vi "frequency estimation special.vi"() -> ()   [LabVIEW 2014]
uses:
  <vilib>/LabVIEW Targets/FPGA/cRIO/shared/nicrio_ModuleControls/nicrio_cRIO-9467_Altitude.ctl
  <vilib>/LabVIEW Targets/FPGA/cRIO/shared/nicrio_ModuleControls/nicrio_cRIO-9467_Longitude.ctl
  <vilib>/LabVIEW Targets/FPGA/cRIO/shared/nicrio_ModuleControls/nicrio_cRIO-9467_Latitude.ctl
  <vilib>/LabVIEW Targets/FPGA/cRIO/shared/nicrio_ModuleControls/nicrio_cRIO-9225_DataRatesRing.ctl
  <vilib>/LabVIEW Targets/FPGA/cRIO/shared/nicrio_ModuleControls/nicrio_cRIO-9227_DataRatesRing.ctl
  <vilib>/Platform/TimedLoop/XDataNode/timing_clust.ctl
  <vilib>/Platform/TimedLoop/XDataNode/nitl_modes.ctl
  <vilib>/Platform/TimedLoop/XDataNode/wakeup.ctl
  <vilib>/rvi/FXPMathLib/FxpSinAndCos/subVIs/nifxpmath_SinAndCos_SimConfig.ctl
  <vilib>/rvi/FXPMathLib/FxpRectToPolar/subVIs/nifxpmath_RectToPolar_SimConfig.ctl
  <vilib>/rvi/Emulation/niFpgaGetClockAttributes.vi
  <vilib>/rvi/Emulation/niFpgaSctlEmulationGetInTimedLoop.vi
  <vilib>/rvi/Emulation/niFpgaEmulationReportErrorSimple.vi
  <vilib>/rvi/eio/common/nirviEmuTemplateMethod_errors.vi
  <vilib>/rvi/eio/common/nirviEmuTemplatePropertyGet_noerrors.vi
  <vilib>/rvi/Emulation/niFpgaCriticalErrorInLSC.vi
  <vilib>/rvi/Memory/Memory_Emulation/nirvimemoryFastEmulation.vi
  <vilib>/rvi/Memory/Memory_Emulation/nirvimemoryEmulation.vi
  <vilib>/rvi/Emulation/niFpgaEmulationIsFPGAContextNoSignature.vi
  <vilib>/rvi/DataTransferAndStorage/Container/Common/niFpgaContainerGetUniqueNameForEmu.vi
  <vilib>/rvi/Emulation/niFpgaProcessEmulError.vi
  <vilib>/rvi/errors/nirviReportUnexpectedCaseInternalError (U32).vi
  <vilib>/rvi/FXPMathLib/FxpSinAndCos/simVIs/DllFxpSinAndCosTemp_sub.vi
  <vilib>/rvi/FXPMathLib/FxpRectToPolar/simVIs/DllFxpRectToPolarTemp_sub.vi
  <vilib>/rvi/interface/RandomDataEmulation/niFpgaRandomDataHandleErrors.vi
  <vilib>/rvi/DataTransferAndStorage/Container/Common/niFpgaContainerSetEmuInfo.vi
  <vilib>/rvi/eio/common/nirviEmuReportErrorAndStop.vi
  <vilib>/rvi/eio/common/nirviEmuTemplatePropertySet_noerrors.vi
  <vilib>/rvi/eio/common/nirviEmuTemplatePropertyGet_errors.vi
  <vilib>/eio/EIOMethodNode/EIOMethodNode.xnode
  <vilib>/eio/EIOPropertyNode/EIOPropertyNode.xnode
  <vilib>/eio/EIONode/EIONode.xnode
  <vilib>/Platform/TimedLoop/XDataNode/XDataNode.xnode
  <vilib>/rvi/DataTransferAndStorage/Container/XNode/niFpgaContainer.xnode
  <vilib>/rvi/FXPMathLib/FxpMul/XNode/nifxpmath_Multiplier.xnode
  <vilib>/rvi/FXPMathLib/FxpSinAndCos/XNode/nifxpmath_SinAndCos.xnode
  <vilib>/rvi/FXPMathLib/FxpAdd/XNode/nifxpmath_Add.xnode
  <vilib>/rvi/FXPMathLib/FxpRectToPolar/XNode/nifxpmath_RectToPolar.xnode
  <vilib>/rvi/interface/RandomDataEmulation/nirviRandomDataFpgaReadWriteTemplate.vi
  <vilib>/rvi/LocalResourceManager/LocalResourceManager.xnode
  <vilib>/rvi/FXPMathLib/sim/FxpSim.dll
  <vilib>/Platform/TimedLoop/XDataNode/XDNodeRunTimeDep.lvlib
  <vilib>/rvi/eio/common/nirviEmuTemplatePropertySet_errors.vi
  akhil/fpga timekeeper/FPGA Timekeeper.lvlib
panel:
  out "Firmware Version":u32 format="%.0x"
  out "Vendor ID":u16 format="%.0x"
  out "Module ID":u16 format="%.0x"
  out "Serial Number":u32 format="%.0x"
  out "FPGA Error Out":errorcluster
  in  "stop 2":bool
  out "PPS Timestamp (TAI)":u64
  out "UTC Offset":i8
  out "UTC Offset Valid":bool
  out "GPS Status":T1(ring)
  out "Antenna Status":T2(ring)
  out "Leap Second Direction":enum8{"Add", "Delete"}(ring)
  out "Leap Second Pending":bool
  out "Leap Second Occurred":bool
  out "Satellites Available":u8
  out "Self-Survey Complete":bool
  out "Latitude (°)":T3 format="%.6f"
  out "Longitude (°)":T4 format="%.6g"
  out "Altitude (m)":T5 format="%.2f"
  out "Timed Out":bool
  out "Iterations":i32
  out "FPGA Timekeeper time (ns)":u64
  out "GPS status":T1(ring)
  out "FPGA Timekeeper locked":bool
  out "offset from time reference":i32
  out "antenna status":T2(ring)
  out "satellites available":u8
  out "UTC offset":i8
  out "UTC offset valid":bool
  out "rate of chage of frequency":fxp<+/-,17,17>
  out "ry phase diff":fxp<+/-,17,17>
  out "phase current":fxp<+/-,17,17>
  out "phase voltage":fxp<+/-,17,17>
  out "current frequency":fxp<+/-,35,18>
  out "voltage frequency":fxp<+/-,35,18>
  out "Array":T6(array[cluster])
  out "theta":fxp<+/-,22,10>[](array[numeric])
  out "r":fxp<+,60,17>[](array[numeric])
  in  "stop":bool
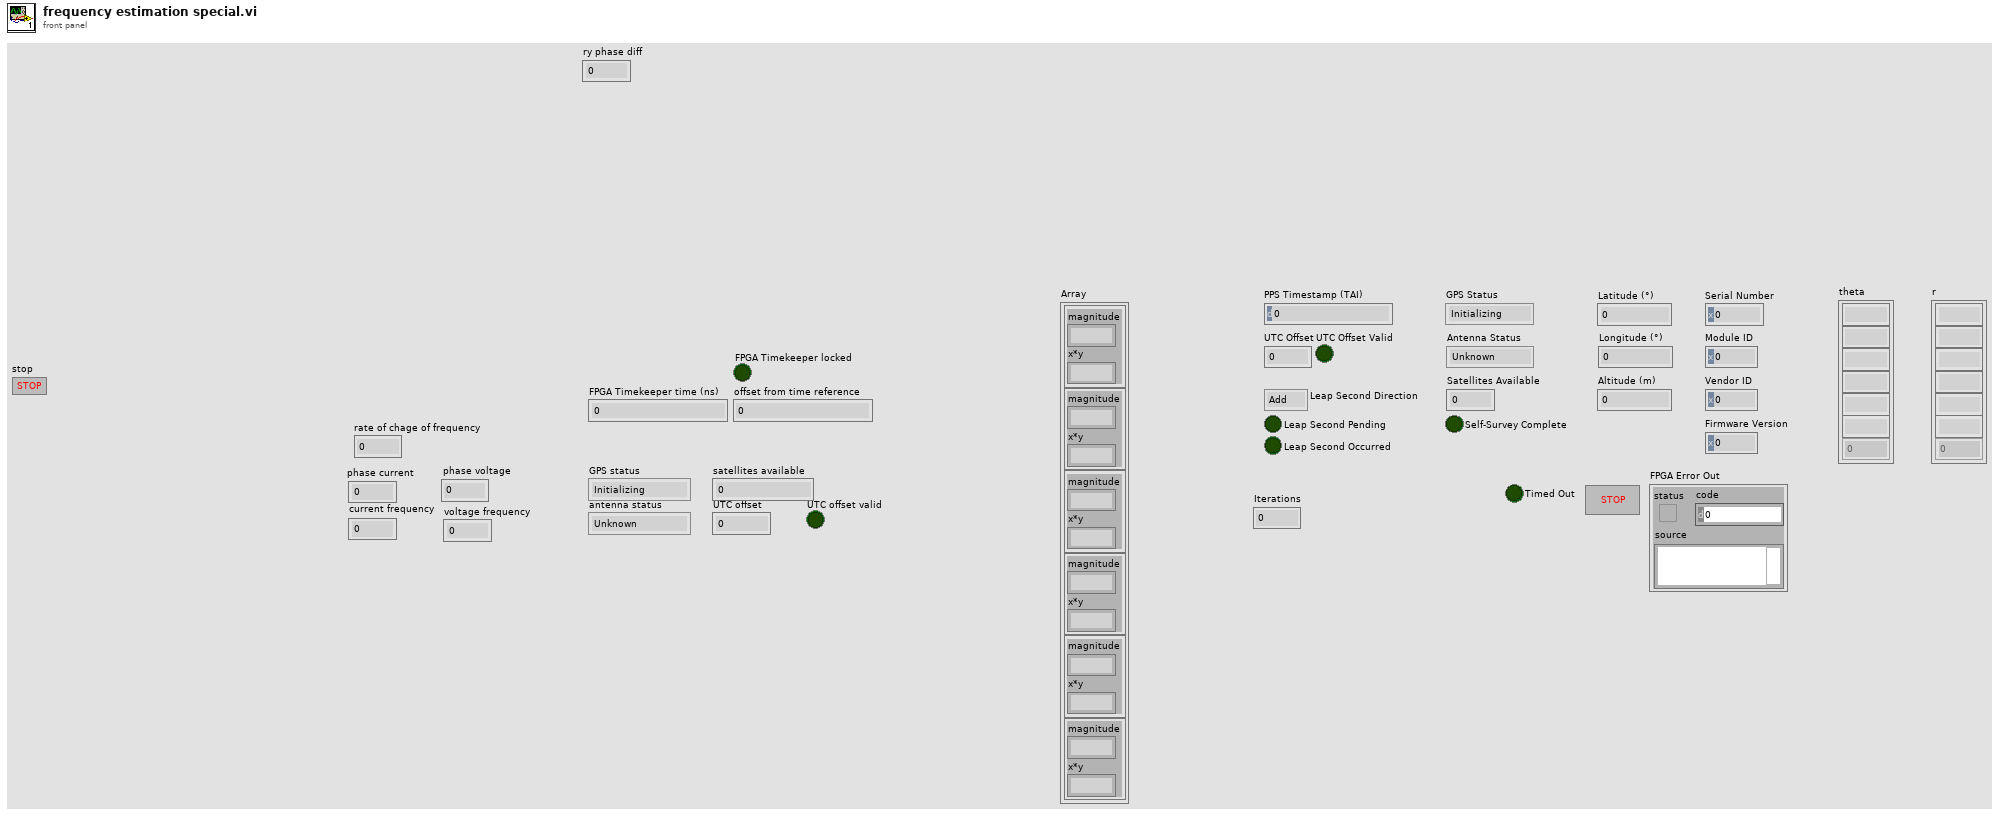
[diagram p1: front panel]
types:
  T1 = enum8{"Initializing", "Normal", "Unable to get fix"}
  T2 = enum8{"Unknown", "Normal", "Absent", "Overcurrent"}
  T3 = typedef "nicrio_cRIO-9467_Latitude.ctl" = fxp<+/-,28,8>
  T4 = typedef "nicrio_cRIO-9467_Longitude.ctl" = fxp<+/-,29,9>
  T5 = typedef "nicrio_cRIO-9467_Altitude.ctl" = fxp<+/-,24,17>
  T6 = cluster{"magnitude":fxp<+,60,17>, "x*y":fxp<+/-,22,10>}[]
  T7 = typedef "nicrio_cRIO-9227_DataRatesRing.ctl" = u8
  T8 = typedef "nicrio_cRIO-9225_DataRatesRing.ctl" = u8
  T9 = typedef "XDNodeRunTimeDep.lvlib/timing_clust.ctl" = cluster{"Expected End [f-1]":u64, "Actual End [f-1]":u64, "Finished Late? [f-1]":bool, "Expected End [i-1]":u64, "Actual End [i-1]":u64, "Finished Late? [i-1]":bool, "Expected Start [i]":u64, "Actual Start [i]":u64, "Expected Start [f]":u64, "Actual Start [f]":u64, "Source Name":string, "Structure Name":string, "Period":i64, "Deadline":i64, "Offset":i64, "Start":i64, "Priority":i32, "Timeout":i32, "Mode":T10, "Wakeup Reason":T11, "Error":errorcluster, "Source Type":string, "Secondary Source Type":string, "Global End Time":u64, "Global Start Time":u64, "Frame Duration":u64, "Iteration Duration":u64, "Assigned CPU":i32, "I/O Scan Engine Mode":u32}
  T10 = typedef "XDNodeRunTimeDep.lvlib/nitl_modes.ctl" = enum32{"No Change", "Process missed periods, maintain original phase", "Discard missed periods, maintain original phase", "Process missed periods, ignore original phase", "Discard missed periods, ignore original phase"}
  T11 = typedef "XDNodeRunTimeDep.lvlib/wakeup.ctl" = enum32{"Normal", "Aborted", "Asynchronous wakeup", "Timing source error", "Timed loop error", "Timeout"}
  T12 = cluster{"magnitude":fxp<+,60,17>, "x*y":fxp<+/-,22,10>}
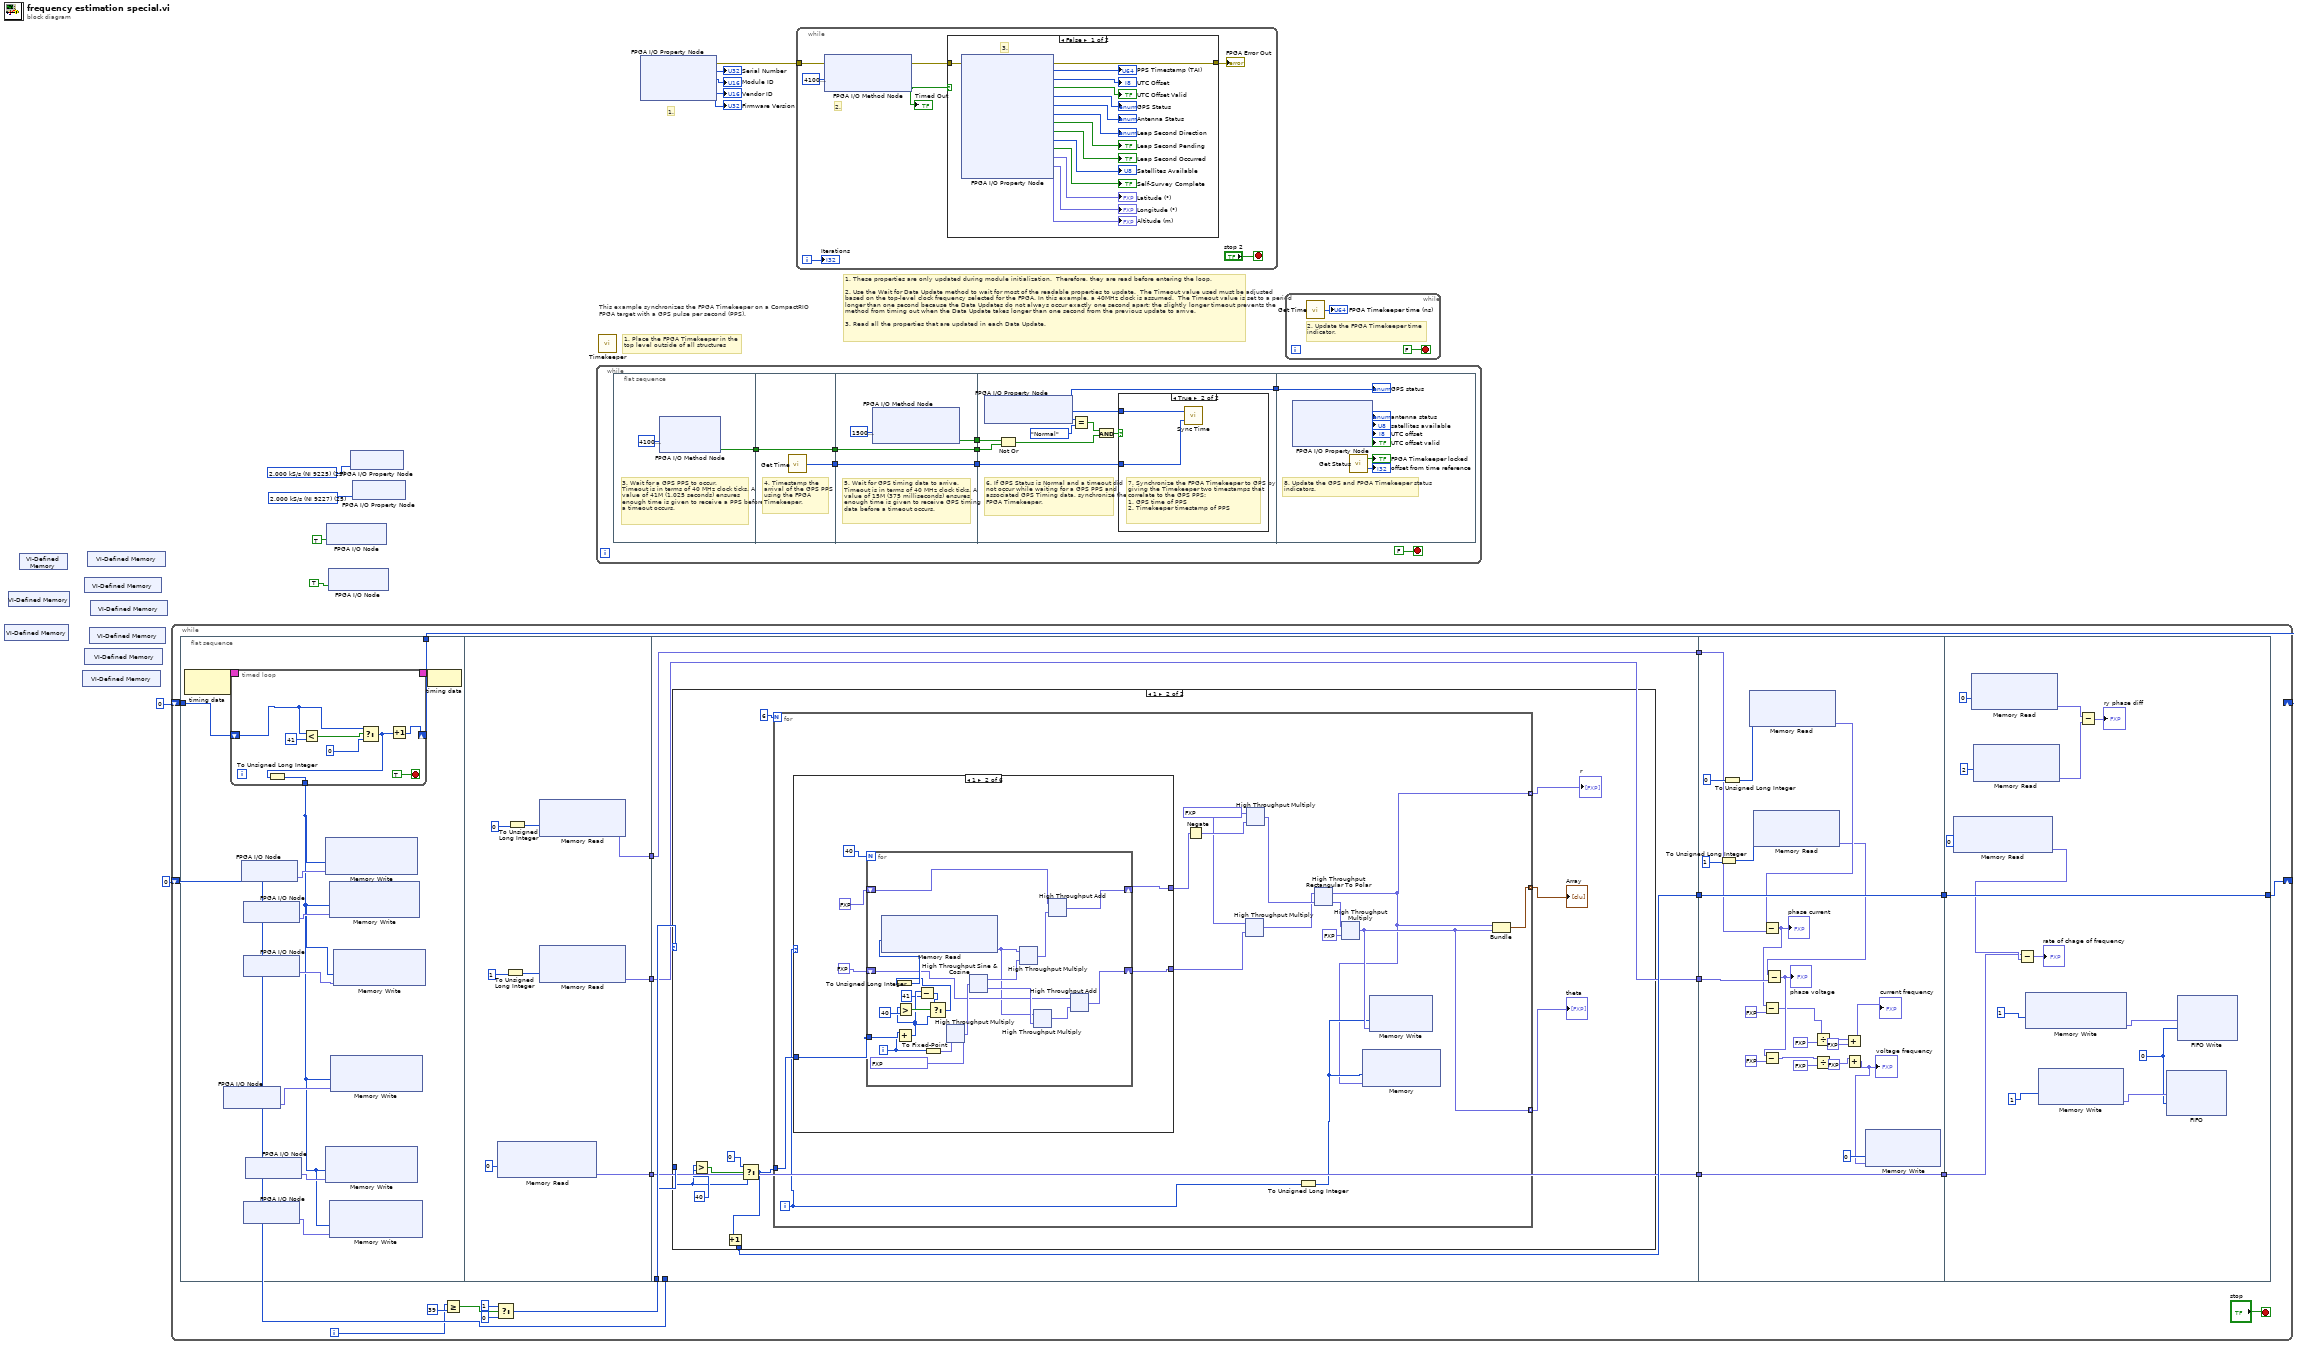
[diagram p0: block diagram]
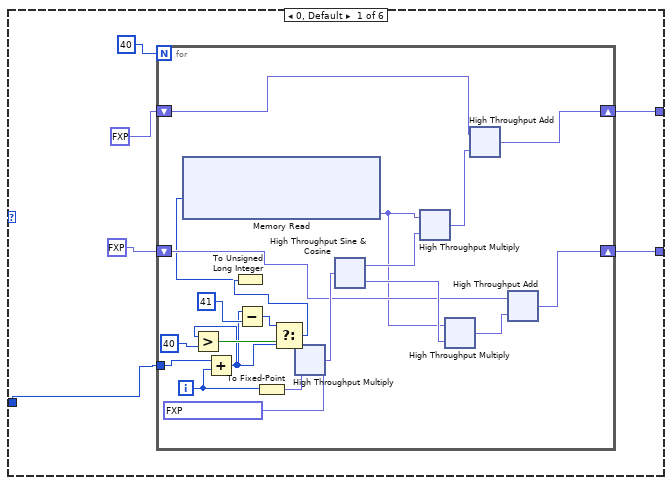
[diagram p5: hidden frame]
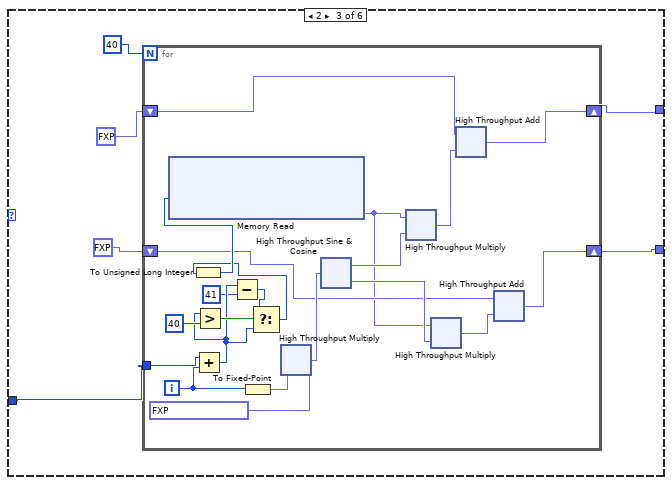
[diagram p6: hidden frame]
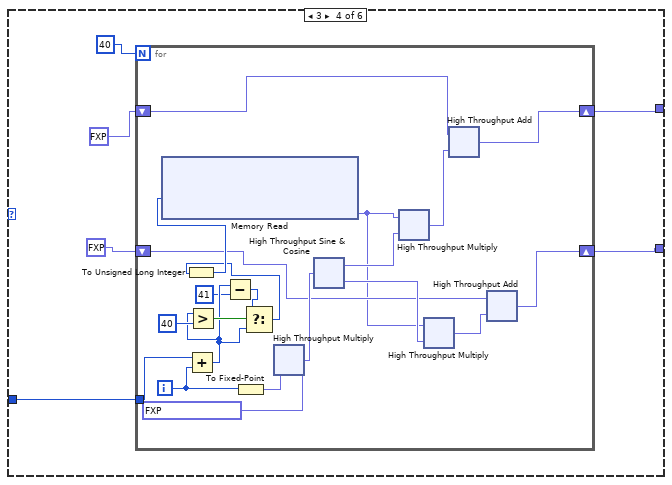
[diagram p7: hidden frame]
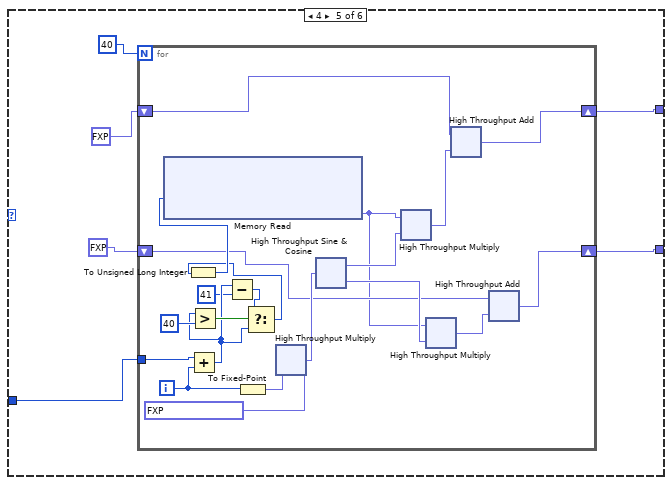
[diagram p8: hidden frame]
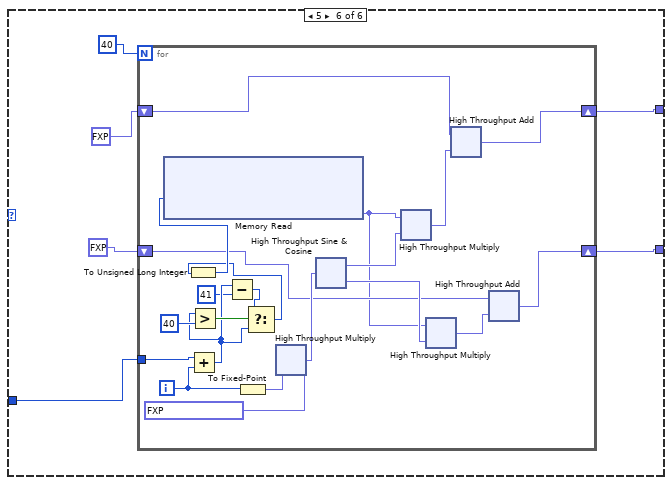
[diagram p9: hidden frame]
diagram:
  w9 = T7 25 items=["50.000 kS/s (NI 9227)"=1, "25.000 kS/s (NI 9227)"=2, "16.667 kS/s (NI 9227)"=3, "12.500 kS/s (NI 9227)"=4, "10.000 kS/s (NI 9227)"=5, "8.333 kS/s (NI 9227)"=6, "7.143 kS/s (NI 9227)"=7, "6.250 kS/s (NI 9227)"=8, "5.556 kS/s (NI 9227)"=9, "5.000 kS/s (NI 9227)"=10, "4.545 kS/s (NI 9227)"=11, "4.167 kS/s (NI 9227)"=12, "3.846 kS/s (NI 9227)"=13, "3.571 kS/s (NI 9227)"=14, "3.333 kS/s (NI 9227)"=15, "3.125 kS/s (NI 9227)"=16, "2.941 kS/s (NI 9227)"=17, "2.778 kS/s (NI 9227)"=18, "2.632 kS/s (NI 9227)"=19, "2.500 kS/s (NI 9227)"=20, "2.381 kS/s (NI 9227)"=21, "2.273 kS/s (NI 9227)"=22, "2.174 kS/s (NI 9227)"=23, "2.083 kS/s (NI 9227)"=24, "2.000 kS/s (NI 9227)"=25, "1.923 kS/s (NI 9227)"=26, "1.852 kS/s (NI 9227)"=27, "1.786 kS/s (NI 9227)"=28, "1.724 kS/s (NI 9227)"=29, "1.667 kS/s (NI 9227)"=30, "1.613 kS/s (NI 9227)"=31] ("Data Rate")
  w6 = T8 25 items=["50.000 kS/s (NI 9225)"=1, "25.000 kS/s (NI 9225)"=2, "16.667 kS/s (NI 9225)"=3, "12.500 kS/s (NI 9225)"=4, "10.000 kS/s (NI 9225)"=5, "8.333 kS/s (NI 9225)"=6, "7.143 kS/s (NI 9225)"=7, "6.250 kS/s (NI 9225)"=8, "5.556 kS/s (NI 9225)"=9, "5.000 kS/s (NI 9225)"=10, "4.545 kS/s (NI 9225)"=11, "4.167 kS/s (NI 9225)"=12, "3.846 kS/s (NI 9225)"=13, "3.571 kS/s (NI 9225)"=14, "3.333 kS/s (NI 9225)"=15, "3.125 kS/s (NI 9225)"=16, "2.941 kS/s (NI 9225)"=17, "2.778 kS/s (NI 9225)"=18, "2.632 kS/s (NI 9225)"=19, "2.500 kS/s (NI 9225)"=20, "2.381 kS/s (NI 9225)"=21, "2.273 kS/s (NI 9225)"=22, "2.174 kS/s (NI 9225)"=23, "2.083 kS/s (NI 9225)"=24, "2.000 kS/s (NI 9225)"=25, "1.923 kS/s (NI 9225)"=26, "1.852 kS/s (NI 9225)"=27, "1.786 kS/s (NI 9225)"=28, "1.724 kS/s (NI 9225)"=29, "1.667 kS/s (NI 9225)"=30, "1.613 kS/s (NI 9225)"=31] ("Data Rate")
  # "1."
  # "1. These properties are only updated during module initialization.  Therefore, they are read before entering the loop.\n\n2. Use the Wait for Data Update method to wait for most of the readable properties to update.  The Timeout value used must be adjusted based on the top-level clock frequency selected for the FPGA. In this example, a 40MHz clock is assumed.  The Timeout value is set to a period longer than one second because the Data Updates do not always occur exactly one second apart; the slightly longer timeout prevents the method from timing out when the Data Update takes longer than one second from the previous update to arrive. \n\n3. Read all the properties that are updated in each Data Update."
  # "This example synchronizes the FPGA Timekeeper on a CompactRIO FPGA target with a GPS pulse per second (PPS)."
  # "1. Place the FPGA Timekeeper in the\ntop level outside of all structures"
  n1 = xnode "VI-Defined Memory"() -> ()  [unwired: 1 out]
  n2 = xnode "VI-Defined Memory"() -> ()  [unwired: 1 out]
  n3 = xnode "VI-Defined Memory"() -> ()  [unwired: 1 out]
  n4 = xnode "VI-Defined Memory"() -> ()  [unwired: 1 out]
  n5 = xnode "VI-Defined Memory"() -> ()  [unwired: 1 out]
  n6 = xnode "VI-Defined Memory"() -> ()  [unwired: 1 out]
  n7 = xnode "VI-Defined Memory"() -> ()  [unwired: 1 out]
  n8 = xnode "VI-Defined Memory"() -> ()  [unwired: 1 out]
  n9 = xnode "VI-Defined Memory"() -> ()  [unwired: 1 out]
  n10 = while {
    shift-right: [w29] -> _
    shift-left: i16 0 -> [w30]
    shift-right: [w22] -> _
    shift-left: u32 0 ("t") -> [w23]
    i -> [w21]
    stop <- "stop" stop-if-true
    n11 = flat-sequence {
      tunnel: w30 -> [w41]
      tunnel: [w40] -> w29
      tunnel: [w58] -> w20
      tunnel: [w57] -> w19
      tunnel: [w55] -> w16
      tunnel: w24 -> [w68]
      tunnel: w23 -> [w67]
      tunnel: [w66] -> w15
      tunnel: w20 -> [w65]
      tunnel: [w65] -> w14
      tunnel: [w64] -> w13
      tunnel: w19 -> [w64]
      tunnel: [w63] -> w12
      tunnel: w16 -> [w63]
      tunnel: w15 -> [w497]
      tunnel: w14 -> [w492]
      tunnel: w13 -> [w491]
      tunnel: [w497] -> w18
      tunnel: [w473] -> w17
      tunnel: w12 -> [w473]
      tunnel: [w512] -> w22
      tunnel: w18 -> [w512]
      tunnel: w17 -> [w510]
      frame #0 {
        n12 = node-c288() -> (w33:T9)  [unwired: 1 in]
        n13 = xnode "FPGA I/O Node"() -> ("Mod1/AI1"=w42:fxp<+/-,24,10>)  [unwired: 1 in, 1 out]
        n14 = timed-loop {
          timing: w33 -> [_]
          timing-out: [_] -> w32
          tunnel: [w44] -> w34
          shift-right: [w45] -> w40
          shift-left: w41 -> [w46]
          stop <- TRUE stop-if-true
          n15 = Less?(x=w46, y=i16 41) -> (x < y?=w49:bool)
          n16 = Select(t=w46, s=w49, f=i16 0) -> (s? t:f=w47:i16)
          n17 = To Unsigned Long Integer(number=w47) -> (unsigned 32bit integer=w44:u32)
          n18 = Increment(x=w47) -> (x+1=w45:i16)
        }
        n19 = xnode "FPGA I/O Node"() -> ("Mod2/AI1"=w39:fxp<+/-,24,5>)  [unwired: 1 in, 1 out]
        n20 = xnode "FPGA I/O Node"() -> ("Mod2/AI0"=w36:fxp<+/-,24,5>)  [unwired: 1 in, 1 out]
        n21 = xnode "FPGA I/O Node"() -> ("Mod1/AI2"=w37:fxp<+/-,24,10>)  [unwired: 1 in, 1 out]
        n22 = xnode "FPGA I/O Node"() -> ("Mod2/AI2"=w35:fxp<+/-,24,5>)  [unwired: 1 in, 1 out]
        n23 = xnode "FPGA I/O Node"() -> ("Mod1/AI0"=w38:fxp<+/-,24,10>)  [unwired: 1 in, 1 out]
        n24 = xnode ("Memory Write")("Address"=w34, "Data"=w39) -> ()  [unwired: 1 in, 1 out]
        n25 = xnode ("Memory Write")("Address"=w34, "Data"=w38) -> ()  [unwired: 1 in, 1 out]
        n26 = xnode ("Memory Write")("Address"=w34, "Data"=w36) -> ()  [unwired: 1 in, 1 out]
        n27 = xnode ("Memory Write")("Address"=w34, "Data"=w37) -> ()  [unwired: 1 in, 1 out]
        n28 = xnode ("Memory Write")("Address"=w34, "Data"=w42) -> ()  [unwired: 1 in, 1 out]
        n29 = xnode ("Memory Write")("Address"=w34, "Data"=w35) -> ()  [unwired: 1 in, 1 out]
        n30 = node-c288(w32) -> ()
      }
      frame #1 {
        n31 = xnode ("Memory Read")("Address"=u32 0) -> ("Data"=w55:fxp<+/-,16,16>)  [unwired: 1 in, 1 out]
        n32 = To Unsigned Long Integer(number=i16 1) -> (unsigned 32bit integer=w59:u32)
        n33 = To Unsigned Long Integer(number=i16 0) -> (unsigned 32bit integer=w61:u32)
        n34 = xnode ("Memory Read")("Address"=w61) -> ("Data"=w58:fxp<+/-,16,16>)  [unwired: 1 in, 1 out]
        n35 = xnode ("Memory Read")("Address"=w59) -> ("Data"=w57:fxp<+/-,16,16>)  [unwired: 1 in, 1 out]
      }
      frame #2 {
        n36 = case shown="1" w68 {
          tunnel: w67 -> [w69 w75]
          tunnel: [w69 w78] -> w66
          frame 0, Default {
          }
          frame 1 {
            n37 = Greater?(x=w75, y=u32 40) -> (0:w76:bool)
            n38 = Select(t=u32 0, s=w76, f=w75) -> (s? t:f=w73:u32)
            n39 = Increment(x=w73) -> (x+1=w78:u32)
            n40 = for {
              N: 6 -> [_]
              tunnel: w73 -> [w86]
              tunnel: [w83] -> w72 mode=indexing
              tunnel: [w82] -> w71 mode=indexing
              tunnel: [w80] -> w70 mode=indexing
              i -> [w84]
              w92 = fxp<+/-,16,1> 0.03533935546875 ("x")
              n41 = case shown="1" w84 {
                tunnel: [w132 w188 w245 w302 w359 w416] -> w87
                tunnel: w86 -> [w131 w190 w247 w304 w361 w418]
                tunnel: [w133 w189 w246 w303 w360 w417] -> w85
                frame 0, Default {
                  n42 = for {
                    N: 40 ("Numeric") -> [_]
                    shift-right: [w150] -> w132
                    shift-left: fxp<+,1,1> 0.0 ("x+y") -> [w149]
                    shift-right: [w153] -> w133
                    shift-left: fxp<+,1,1> 0.0 -> [w148]
                    tunnel: w131 -> [w140]
                    i -> [w141]
                    n43 = Add(x=w140, y=w141) -> (x+y=w139:u32)
                    n44 = Greater?(x=w139, y=u32 40) -> (0:w144:bool)
                    n45 = Subtract(x=w139, y=u32 41) -> (x-y=w142:u32)
                    n46 = To Fixed-Point(number=w141) -> (fixed-point=w157:fxp<+/-,32,32>)  [unwired: 1 in]
                    n47 = Select(t=w142, s=w144, f=w139) -> (s? t:f=w138:u32)
                    n48 = To Unsigned Long Integer(number=w138) -> (unsigned 32bit integer=w137:u32)
                    n49 = xnode ("Memory Read")("Address"=w137) -> ("Data"=w146:fxp<+/-,25,11>)  [unwired: 1 in, 1 out]
                    n50 = xnode ("High Throughput Multiply")("x"=fxp<+/-,32,16> 0.04998779296875 ("number"), "y"=w157) -> ("x*y"=w156:fxp<+/-,64,48>)
                    n51 = xnode "High Throughput Sine & Cosine"("x (pi)"=w156) -> ("sin(x)"=w155:fxp<+/-,16,2>, "cos(x)"=w152:fxp<+/-,16,2>)
                    n52 = xnode ("High Throughput Multiply")("x"=w146, "y"=w155) -> ("x*y"=w154:fxp<+/-,41,13>)
                    n53 = xnode ("High Throughput Multiply")("x"=w146, "y"=w152) -> ("x*y"=w151:fxp<+/-,41,13>)
                    n54 = xnode ("High Throughput Add")("x"=w148, "y"=w154) -> ("x+y"=w153:fxp<+/-,42,14>)
                    n55 = xnode ("High Throughput Add")("x"=w149, "y"=w151) -> ("x+y"=w150:fxp<+/-,44,16>)
                  }
                }
                frame 1 {
                  n56 = for {
                    N: 40 ("Numeric") -> [_]
                    shift-right: [w206] -> w188
                    shift-left: fxp<+,1,1> 0.0 ("x+y") -> [w205]
                    shift-right: [w209] -> w189
                    shift-left: fxp<+,1,1> 0.0 -> [w204]
                    tunnel: w190 -> [w201]
                    i -> [w200]
                    n57 = Add(x=w201, y=w200) -> (x+y=w196:u32)
                    n58 = Greater?(x=w196, y=u32 40) -> (0:w198:bool)
                    n59 = Subtract(x=w196, y=u32 41) -> (x-y=w194:u32)
                    n60 = To Fixed-Point(number=w200) -> (fixed-point=w213:fxp<+/-,32,32>)  [unwired: 1 in]
                    n61 = Select(t=w194, s=w198, f=w196) -> (s? t:f=w197:u32)
                    n62 = To Unsigned Long Integer(number=w197) -> (unsigned 32bit integer=w214:u32)
                    n63 = xnode ("Memory Read")("Address"=w214) -> ("Data"=w202:fxp<+/-,25,11>)  [unwired: 1 in, 1 out]
                    n64 = xnode ("High Throughput Multiply")("x"=fxp<+/-,32,16> 0.04998779296875 ("number"), "y"=w213) -> ("x*y"=w212:fxp<+/-,64,48>)
                    n65 = xnode "High Throughput Sine & Cosine"("x (pi)"=w212) -> ("sin(x)"=w211:fxp<+/-,16,2>, "cos(x)"=w208:fxp<+/-,16,2>)
                    n66 = xnode ("High Throughput Multiply")("x"=w202, "y"=w211) -> ("x*y"=w210:fxp<+/-,41,13>)
                    n67 = xnode ("High Throughput Multiply")("x"=w202, "y"=w208) -> ("x*y"=w207:fxp<+/-,41,13>)
                    n68 = xnode ("High Throughput Add")("x"=w204, "y"=w210) -> ("x+y"=w209:fxp<+/-,42,14>)
                    n69 = xnode ("High Throughput Add")("x"=w205, "y"=w207) -> ("x+y"=w206:fxp<+/-,44,16>)
                  }
                }
                frame 2 {
                  n70 = for {
                    N: 40 ("Numeric") -> [_]
                    shift-right: [w263] -> w245
                    shift-left: fxp<+,1,1> 0.0 ("x+y") -> [w262]
                    shift-right: [w266] -> w246
                    shift-left: fxp<+,1,1> 0.0 -> [w261]
                    tunnel: w247 -> [w258]
                    i -> [w257]
                    n71 = Add(x=w258, y=w257) -> (x+y=w253:u32)
                    n72 = Greater?(x=w253, y=u32 40) -> (0:w255:bool)
                    n73 = Subtract(x=w253, y=u32 41) -> (x-y=w251:u32)
                    n74 = To Fixed-Point(number=w257) -> (fixed-point=w270:fxp<+/-,32,32>)  [unwired: 1 in]
                    n75 = Select(t=w251, s=w255, f=w253) -> (s? t:f=w254:u32)
                    n76 = To Unsigned Long Integer(number=w254) -> (unsigned 32bit integer=w271:u32)
                    n77 = xnode ("Memory Read")("Address"=w271) -> ("Data"=w259:fxp<+/-,25,11>)  [unwired: 1 in, 1 out]
                    n78 = xnode ("High Throughput Multiply")("x"=fxp<+/-,32,16> 0.04998779296875 ("number"), "y"=w270) -> ("x*y"=w269:fxp<+/-,64,48>)
                    n79 = xnode "High Throughput Sine & Cosine"("x (pi)"=w269) -> ("sin(x)"=w268:fxp<+/-,16,2>, "cos(x)"=w265:fxp<+/-,16,2>)
                    n80 = xnode ("High Throughput Multiply")("x"=w259, "y"=w268) -> ("x*y"=w267:fxp<+/-,41,13>)
                    n81 = xnode ("High Throughput Multiply")("x"=w259, "y"=w265) -> ("x*y"=w264:fxp<+/-,41,13>)
                    n82 = xnode ("High Throughput Add")("x"=w261, "y"=w267) -> ("x+y"=w266:fxp<+/-,42,14>)
                    n83 = xnode ("High Throughput Add")("x"=w262, "y"=w264) -> ("x+y"=w263:fxp<+/-,44,16>)
                  }
                }
                frame 3 {
                  n84 = for {
                    N: 40 ("Numeric") -> [_]
                    shift-right: [w320] -> w302
                    shift-left: fxp<+,1,1> 0.0 ("x+y") -> [w319]
                    shift-right: [w323] -> w303
                    shift-left: fxp<+,1,1> 0.0 -> [w318]
                    tunnel: w304 -> [w308]
                    i -> [w315]
                    n85 = Add(x=w308, y=w315) -> (x+y=w311:u32)
                    n86 = Greater?(x=w311, y=u32 40) -> (0:w313:bool)
                    n87 = Subtract(x=w311, y=u32 41) -> (x-y=w309:u32)
                    n88 = To Fixed-Point(number=w315) -> (fixed-point=w327:fxp<+/-,32,32>)  [unwired: 1 in]
                    n89 = Select(t=w309, s=w313, f=w311) -> (s? t:f=w312:u32)
                    n90 = To Unsigned Long Integer(number=w312) -> (unsigned 32bit integer=w328:u32)
                    n91 = xnode ("Memory Read")("Address"=w328) -> ("Data"=w316:fxp<+/-,25,11>)  [unwired: 1 in, 1 out]
                    n92 = xnode ("High Throughput Multiply")("x"=fxp<+/-,32,16> 0.04998779296875 ("number"), "y"=w327) -> ("x*y"=w326:fxp<+/-,64,48>)
                    n93 = xnode "High Throughput Sine & Cosine"("x (pi)"=w326) -> ("sin(x)"=w325:fxp<+/-,16,2>, "cos(x)"=w322:fxp<+/-,16,2>)
                    n94 = xnode ("High Throughput Multiply")("x"=w316, "y"=w325) -> ("x*y"=w324:fxp<+/-,41,13>)
                    n95 = xnode ("High Throughput Multiply")("x"=w316, "y"=w322) -> ("x*y"=w321:fxp<+/-,41,13>)
                    n96 = xnode ("High Throughput Add")("x"=w318, "y"=w324) -> ("x+y"=w323:fxp<+/-,42,14>)
                    n97 = xnode ("High Throughput Add")("x"=w319, "y"=w321) -> ("x+y"=w320:fxp<+/-,44,16>)
                  }
                }
                frame 4 {
                  n98 = for {
                    N: 40 ("Numeric") -> [_]
                    shift-right: [w377] -> w359
                    shift-left: fxp<+,1,1> 0.0 ("x+y") -> [w376]
                    shift-right: [w380] -> w360
                    shift-left: fxp<+,1,1> 0.0 -> [w375]
                    tunnel: w361 -> [w365]
                    i -> [w372]
                    n99 = Add(x=w365, y=w372) -> (x+y=w368:u32)
                    n100 = Greater?(x=w368, y=u32 40) -> (0:w370:bool)
                    n101 = Subtract(x=w368, y=u32 41) -> (x-y=w366:u32)
                    n102 = To Fixed-Point(number=w372) -> (fixed-point=w384:fxp<+/-,32,32>)  [unwired: 1 in]
                    n103 = Select(t=w366, s=w370, f=w368) -> (s? t:f=w369:u32)
                    n104 = To Unsigned Long Integer(number=w369) -> (unsigned 32bit integer=w385:u32)
                    n105 = xnode ("Memory Read")("Address"=w385) -> ("Data"=w373:fxp<+/-,25,11>)  [unwired: 1 in, 1 out]
                    n106 = xnode ("High Throughput Multiply")("x"=fxp<+/-,32,16> 0.04998779296875 ("number"), "y"=w384) -> ("x*y"=w383:fxp<+/-,64,48>)
                    n107 = xnode "High Throughput Sine & Cosine"("x (pi)"=w383) -> ("sin(x)"=w382:fxp<+/-,16,2>, "cos(x)"=w379:fxp<+/-,16,2>)
                    n108 = xnode ("High Throughput Multiply")("x"=w373, "y"=w382) -> ("x*y"=w381:fxp<+/-,41,13>)
                    n109 = xnode ("High Throughput Multiply")("x"=w373, "y"=w379) -> ("x*y"=w378:fxp<+/-,41,13>)
                    n110 = xnode ("High Throughput Add")("x"=w375, "y"=w381) -> ("x+y"=w380:fxp<+/-,42,14>)
                    n111 = xnode ("High Throughput Add")("x"=w376, "y"=w378) -> ("x+y"=w377:fxp<+/-,44,16>)
                  }
                }
                frame 5 {
                  n112 = for {
                    N: 40 ("Numeric") -> [_]
                    shift-right: [w434] -> w416
                    shift-left: fxp<+,1,1> 0.0 ("x+y") -> [w433]
                    shift-right: [w437] -> w417
                    shift-left: fxp<+,1,1> 0.0 -> [w432]
                    tunnel: w418 -> [w422]
                    i -> [w429]
                    n113 = Add(x=w422, y=w429) -> (x+y=w425:u32)
                    n114 = Greater?(x=w425, y=u32 40) -> (0:w427:bool)
                    n115 = Subtract(x=w425, y=u32 41) -> (x-y=w423:u32)
                    n116 = To Fixed-Point(number=w429) -> (fixed-point=w441:fxp<+/-,32,32>)  [unwired: 1 in]
                    n117 = Select(t=w423, s=w427, f=w425) -> (s? t:f=w426:u32)
                    n118 = To Unsigned Long Integer(number=w426) -> (unsigned 32bit integer=w442:u32)
                    n119 = xnode ("Memory Read")("Address"=w442) -> ("Data"=w430:fxp<+/-,25,11>)  [unwired: 1 in, 1 out]
                    n120 = xnode ("High Throughput Multiply")("x"=fxp<+/-,32,16> 0.04998779296875 ("number"), "y"=w441) -> ("x*y"=w440:fxp<+/-,64,48>)
                    n121 = xnode "High Throughput Sine & Cosine"("x (pi)"=w440) -> ("sin(x)"=w439:fxp<+/-,16,2>, "cos(x)"=w436:fxp<+/-,16,2>)
                    n122 = xnode ("High Throughput Multiply")("x"=w430, "y"=w439) -> ("x*y"=w438:fxp<+/-,41,13>)
                    n123 = xnode ("High Throughput Multiply")("x"=w430, "y"=w436) -> ("x*y"=w435:fxp<+/-,41,13>)
                    n124 = xnode ("High Throughput Add")("x"=w432, "y"=w438) -> ("x+y"=w437:fxp<+/-,42,14>)
                    n125 = xnode ("High Throughput Add")("x"=w433, "y"=w435) -> ("x+y"=w434:fxp<+/-,44,16>)
                  }
                }
              }
              n126 = Negate(x=w85) -> (-x=w93:fxp<+/-,43,15>)
              n127 = xnode ("High Throughput Multiply")("x"=w92, "y"=w87) -> ("x*y"=w88:fxp<+/-,60,17>)
              n128 = xnode ("High Throughput Multiply")("x"=w92, "y"=w93) -> ("x*y"=w89:fxp<+/-,59,16>)
              n129 = To Unsigned Long Integer(number=w84) -> (unsigned 32bit integer=w81:u32)
              n130 = xnode "High Throughput Rectangular To Polar"("x"=w88, "y"=w89) -> ("magnitude"=w80:fxp<+,60,17>, "phase (pi)"=w91:fxp<+/-,16,2>)
              n131 = xnode ("High Throughput Multiply")("x"=w91, "y"=fxp<+,6,8> 180.0) -> ("x*y"=w82:fxp<+/-,22,10>)
              n132 = xnode "Memory"("Address"=w81, "Data"=w80) -> ()  [unwired: 1 in, 1 out]
              n133 = xnode ("Memory Write")("Address"=w81, "Data"=w82) -> ()  [unwired: 1 in, 1 out]
              n134 = Bundle("magnitude"=w80, "x*y"=w82) -> (w83:T12)  [unwired: 1 in]
            }
            "Array" <- w72
            "theta" <- w71
            "r" <- w70
          }
        }
      }
      frame #3 {
        n135 = To Unsigned Long Integer(number=i16 1) -> (unsigned 32bit integer=w493:u32)
        n136 = To Unsigned Long Integer(number=i16 0) -> (unsigned 32bit integer=w495:u32)
        n137 = xnode ("Memory Read")("Address"=w495) -> ("Data"=w490:fxp<+/-,16,16>)  [unwired: 1 in, 1 out]
        n138 = xnode ("Memory Read")("Address"=w493) -> ("Data"=w489:fxp<+/-,16,16>)  [unwired: 1 in, 1 out]
        n139 = Subtract(x=w490, y=w492) -> (x-y=w481:fxp<+/-,17,17>)
        "phase current" <- w481
        n140 = Subtract(x=w481, y=fxp<+/-,17,17> 9.0) -> (x-y=w477:fxp<+/-,18,18>)
        n141 = Subtract(x=w489, y=w491) -> (x-y=w479:fxp<+/-,17,17>)
        "phase voltage" <- w479
        n142 = Subtract(x=w479, y=fxp<+/-,17,17> 9.0) -> (x-y=w476:fxp<+/-,18,18>)
        n143 = Divide(x=w477, y=fxp<+/-,17,17> 360.0) -> (x/y=w486:fxp<+/-,35,18>)
        n144 = Divide(x=w476, y=fxp<+/-,17,17> 360.0) -> (x/y=w484:fxp<+/-,35,18>)
        n145 = Add(x=w486, y=fxp<+/-,34,17> 50.0) -> (x+y=→"current frequency":fxp<+/-,36,19>)
        n146 = Add(x=w484, y=fxp<+/-,34,17> 50.0) -> (x+y=w474:fxp<+/-,36,19>)
        "voltage frequency" <- w474
        n147 = xnode ("Memory Write")("Address"=u32 0, "Data"=w474) -> ()  [unwired: 1 in, 1 out]
      }
      frame #4 {
        w500 = i16 0
        n148 = xnode ("Memory Read")("Address"=u32 0) -> ("Data"=w509:fxp<+/-,16,16>)  [unwired: 1 in, 1 out]
        n149 = xnode ("Memory Read")("Address"=u32 0) -> ("Data"=w505:fxp<+/-,16,16>)  [unwired: 1 in, 1 out]
        n150 = xnode ("Memory Read")("Address"=u32 2) -> ("Data"=w504:fxp<+/-,16,16>)  [unwired: 1 in, 1 out]
        n151 = Subtract(x=w509, y=w510) -> (x-y=→"rate of chage of frequency":fxp<+/-,17,17>)
        n152 = xnode ("Memory Write")("Address"=u32 1) -> ("Data"=w502:fxp<+/-,25,11>)  [unwired: 1 in, 1 out]
        n153 = xnode ("Memory Write")("Address"=u32 1) -> ("Data"=w501:fxp<+/-,16,16>)  [unwired: 1 in, 1 out]
        n154 = Subtract(x=w505, y=w504) -> (x-y=→"ry phase diff":fxp<+/-,17,17>)
        n155 = xnode "FIFO"("Element"=w501, "Timeout"=w500) -> ()  [unwired: 1 in, 2 out]
        n156 = xnode "FIFO Write"("Element"=w502, "Timeout"=w500) -> ()  [unwired: 1 in, 2 out]
      }
    }
    n157 = Greater Or Equal?(x=w21, y=39) -> (x >= y?=w27:bool)
    n158 = Select(t=u32 1, s=w27, f=u32 0) -> (s? t:f=w24:u32)
  }
  n159 = xnode "FPGA I/O Node"("Mod1/Start"=TRUE) -> ()  [unwired: 1 in, 1 out]
  n160 = xnode "FPGA I/O Node"("Mod2/Start"=TRUE) -> ()  [unwired: 1 in, 1 out]
  n161 = xnode "FPGA I/O Property Node"("Data Rate"=w6) -> ()  [unwired: 1 in, 1 out]
  n162 = xnode "FPGA I/O Property Node"("Data Rate"=w9) -> ()  [unwired: 1 in, 1 out]
  n163 = while {
    stop <- FALSE stop-if-true
    n164 = flat-sequence {
      tunnel: [w521] -> w519
      tunnel: w519 -> [w524]
      tunnel: [w524] -> w518
      tunnel: [w523] -> w516
      tunnel: [w527] -> w520
      tunnel: w518 -> [w526]
      tunnel: [w526] -> w517
      tunnel: w516 -> [w525]
      tunnel: [w525] -> w515
      tunnel: w520 -> [w536]
      tunnel: w517 -> [w535]
      tunnel: w515 -> [w530]
      tunnel: [w529] -> w514
      tunnel: w514 -> [w546]
      frame #0 {
        # "3. Wait for a GPS PPS to occur.\nTimeout is in terms of 40 MHz clock ticks. A value of 41M (1.025 seconds) ensures enough time is given to receive a PPS before a timeout occurs."
        n165 = xnode "FPGA I/O Method Node"("Timeout"=41000000) -> ("Timed Out"=w521:bool)  [unwired: 1 in, 1 out]
      }
      frame #1 {
        # "4. Timestamp the arrival of the GPS PPS using the FPGA Timekeeper."
        n166 = call "Get Time.vi"() -> ("time (ns)"=w523:u64)
      }
      frame #2 {
        # "5. Wait for GPS timing data to arrive.\nTimeout is in terms of 40 MHz clock ticks. A value of 15M (375 milliseconds) ensures enough time is given to receive GPS timing data before a timeout occurs."
        n167 = xnode "FPGA I/O Method Node"("Timeout"=15000000) -> ("Timed Out"=w527:bool)  [unwired: 1 in, 1 out]
      }
      frame #3 {
        # "6. If GPS Status is Normal and a timeout did not occur while waiting for a GPS PPS and associated GPS Timing data, synchronize the FPGA Timekeeper."
        n168 = xnode "FPGA I/O Property Node"() -> ("PPS Timestamp (TAI)"=w531:u64, "GPS Status"=w529:T1)  [unwired: 1 in, 1 out]
        n169 = Not Or(1:w535, 2:w536) -> (0:w533:bool)
        n170 = Equal?(x=w529, y=T1."Normal") -> (x = y?=w534:bool)
        n171 = And(x=w534, y=w533) -> (x .and. y?=w532:bool)
        n172 = case shown="True" w532 {
          tunnel: w531 -> [_ w539]
          tunnel: w530 -> [_ w538]
          frame False {
          }
          frame True {
            # "7. Synchronize the FPGA Timekeeper to GPS by giving the Timekeeper two timestamps that correlate to the GPS PPS:\n1. GPS time of PPS\n2. Timekeeper timestamp of PPS"
            n173 = call "Sync Time.vi"("FPGA Timekeeper time (ns)"=w538, "time reference time (ns)"=w539) -> ()
          }
        }
      }
      frame #4 {
        # "8. Update the GPS and FPGA Timekeeper status indicators."
        n174 = xnode "FPGA I/O Property Node"() -> ("Antenna Status"=→"antenna status":T2, "Satellites Available"=→"satellites available":u8, "UTC Offset"=→"UTC offset":i8, "UTC Offset Valid"=→"UTC offset valid":bool)  [unwired: 1 in, 1 out]
        n175 = call "Get Status.vi"() -> ("FPGA Timekeeper locked"=→"FPGA Timekeeper locked":bool, "offset from time reference"=→"offset from time reference":i32)
        "GPS status" <- w546
      }
    }
  }
  n176 = call "Timekeeper.vi"() -> ()  [unwired: 12 in]
  n177 = xnode "FPGA I/O Property Node"() -> ("error out"=w1:errorcluster, "Serial Number"=→"Serial Number":u32, "Module ID"=→"Module ID":u16, "Vendor ID"=→"Vendor ID":u16, "Firmware Version"=→"Firmware Version":u32)  [unwired: 2 in, 1 out]
  n178 = while {
    tunnel: w1 -> [w548]
    i -> [w547]
    stop <- "stop 2" stop-if-true
    # "2."
    n179 = xnode "FPGA I/O Method Node"("error in"=w548, "Timeout"=41000000) -> ("error out"=w553:errorcluster, "Timed Out"=w550:bool)  [unwired: 1 in, 1 out]
    "Timed Out" <- w550
    n180 = case shown="False" w550 {
      tunnel: w553 -> [w568 w569]
      tunnel: [w557 w569] -> w552
      frame False {
        # "3."
        n181 = xnode "FPGA I/O Property Node"("error in"=w568) -> ("error out"=w557:errorcluster, "PPS Timestamp (TAI)"=→"PPS Timestamp (TAI)":u64, "UTC Offset"=→"UTC Offset":i8, "UTC Offset Valid"=→"UTC Offset Valid":bool, "GPS Status"=→"GPS Status":T1, "Antenna Status"=→"Antenna Status":T2, "Leap Second Direction"=→"Leap Second Direction":enum8{"Add", "Delete"}, "Leap Second Pending"=→"Leap Second Pending":bool, "Leap Second Occurred"=→"Leap Second Occurred":bool, "Satellites Available"=→"Satellites Available":u8, "Self-Survey Complete"=→"Self-Survey Complete":bool, "Latitude (°)"=→"Latitude (°)":T3, "Longitude (°)"=→"Longitude (°)":T4, "Altitude (m)"=→"Altitude (m)":T5)  [unwired: 1 in, 1 out]
      }
      frame True {
      }
    }
    "FPGA Error Out" <- w552
    "Iterations" <- w547
  }
  n182 = while {
    stop <- FALSE stop-if-true
    # "2. Update the FPGA Timekeeper time indicator."
    n183 = call "Get Time.vi"() -> ("time (ns)"=→"FPGA Timekeeper time (ns)":u64)
  }
